vi "Upload.vi"(8 "error in (no error)":errorcluster, 10 "File":path, 11 "TCP_Client in":refnum<class "TCP_Client.lvclass">) -> (0 "error out":errorcluster, 3 "TCP_Client out":refnum<class "TCP_Client.lvclass">)   [LabVIEW 2023, in "TCP_Client.lvlib" / "TCP_Client.lvclass"]
uses:
  TCP_Client.lvclass
  C:/Program Files (x86)/National Instruments/LabVIEW 2023/vi.lib/ActorFramework/Actor/Actor.lvclass
  <vilib>/ActorFramework/Actor/Actor.lvclass/Actor.ctl
  <vilib>/ActorFramework/Message Enqueuer/Message Enqueuer.lvclass/Message Enqueuer.ctl
  TCP_Client.lvclass/TCP_Client.ctl
  TCP_Client Messages/SendMessageToServer Msg/SendMessageToServer Msg.lvclass/SendMessageToServer Msg.ctl
  <vilib>/ActorFramework/Message Enqueuer/Init from Existing Queue.vi
  <vilib>/ActorFramework/Message Enqueuer/Enqueue.vi
  TCP_Client Messages/SendMessageToServer Msg/SendMessageToServer Msg.lvclass
  C:/Program Files (x86)/National Instruments/LabVIEW 2023/vi.lib/ActorFramework/Message/Message.lvclass
  <vilib>/ActorFramework/Message Priority Queue/Priority Enqueue.vi
  <vilib>/ActorFramework/Message Enqueuer/Message Enqueuer.lvclass
  <vilib>/ActorFramework/Actor/Actor.lvclass
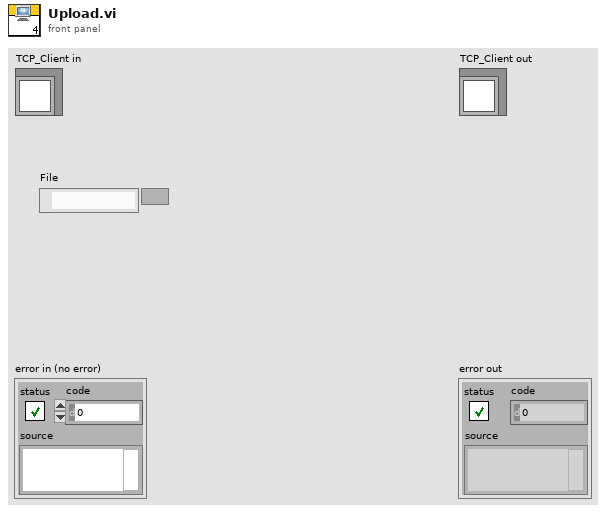
[diagram p1: front panel]
types:
  T1 = enum16{"open", "replace", "create", "open or create", "replace or create", "replace or create with confirmation"}
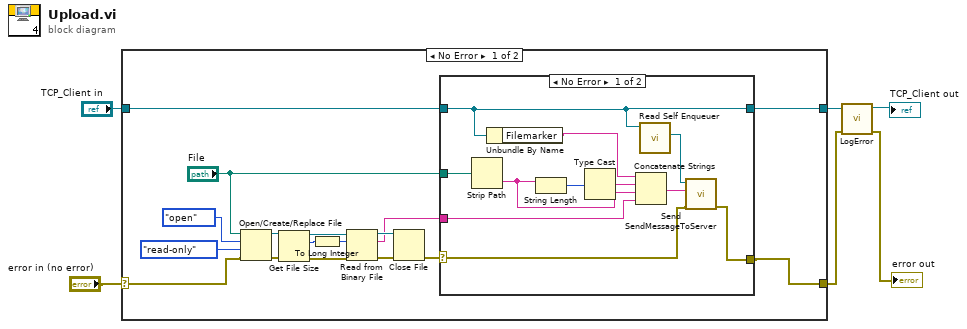
[diagram p0: block diagram]
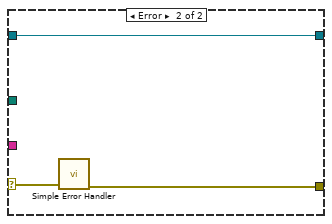
[diagram p2: hidden frame]
diagram:
  n1 = case shown="No Error" "error in (no error)" {
    selector: "error in (no error)" -> [w21 w39]
    tunnel: [w13 w39] -> w2
    tunnel: [w14 w38] -> w4
    tunnel: "TCP_Client in" -> [w15 w38]
    frame No Error {
      n2 = Open/Create/Replace File(file path (use dialog)="File", error in=w21, operation (0:open)=T1."open", access (0:read/write)=enum16{"read/write", "read-only", "write-only"}."read-only") -> (refnum out=w12:refnum<file>, error out=w11:errorcluster)  [unwired: 2 in, 1 out]
      n3 = Get File Size(file=w12, error in=w11) -> (refnum out=w10:refnum<file>, size (in bytes)=w8:i64, 0:w9:errorcluster)
      n4 = To Long Integer(number=w8) -> (32bit integer=w7:i32)
      n5 = Read from Binary File(8:w9, 10:w7, 11:w10) -> (0:w20:errorcluster, 2:w17:string, 3:w19:refnum<file>)  [unwired: 3 in, 1 out]
      n6 = Close File(refnum=w19, error in=w20) -> (error out=w18:errorcluster)  [unwired: 1 out]
      n7 = case shown="No Error" w18 {
        selector: w18 -> [w27 w37]
        tunnel: w17 -> [w31 _]
        tunnel: "File" -> [w30 _]
        tunnel: w15 -> [w25 w35]
        tunnel: [w25 w35] -> w14
        tunnel: [w26 w36] -> w13
        frame No Error {
          n8 = Strip Path(path=w30) -> (name=w34:string)  [unwired: 1 out]
          n9 = Unbundle By Name(w25) -> ("Filemarker"=w24:string)
          n10 = String Length(string=w34) -> (length=w32:i32)
          n11 = Type Cast(x=w32) -> (*(type *) &x=w33:string)  [unwired: 1 in]
          n12 = Concatenate Strings(w24, w33, w34, w31) -> (w28:string)
          n13 = call <vilib>:"Read Self Enqueuer.vi"("Actor"=w25) -> ("Self Enqueuer"=w29:refnum<class "Message Enqueuer.lvclass">)  [unwired: 10 in]
          n14 = call "Send SendMessageToServer.vi"("error in (no error)"=w27, "Message"=w28, "Message Enqueuer"=w29) -> ("error out"=w26:errorcluster)  [unwired: 7 in, 1 out]
        }
        frame Error {
          n15 = call <vilib>:"Simple Error Handler.vi"("error in (no error)"=w37) -> ("error out"=w36:errorcluster)  [unwired: 4 in, 4 out]
        }
      }
    }
    frame Error {
    }
  }
  n16 = call "LogError.vi"("error in (no error)"=w2, "TCP_Client in"=w4) -> ("error out"=→"error out":errorcluster, "TCP_Client out"=→"TCP_Client out":refnum<class "TCP_Client.lvclass">)  [unwired: 8 in]
